vi "Add Package to Feed.vi"(4 "create new package destination folderpath if none exists (F)":bool, 6 "package destination folderpath":path, 7 "create new feed if none exists (F)":bool, 8 "error in":errorcluster, 9 "overwrite existing package (T)":bool=TRUE, 10 "package source filepath":path, 11 "feed folderpath in":path) -> (0 "error out":errorcluster, 2 "package destination filepath":path, 3 "feed folderpath out":path)   [LabVIEW 2014, in "NIPM_API.lvlib"]
doc: "Adds a package to a feed\n\nINPUT(s)\n<B>Feed folderpath</B>: Specifies the folder containing the feed\n\n<B>Package source filepath</B>: Specifies the source filepath of the package to be added to the feed\n\n<B>Create new feed if none exists</B>: If this input is set to TRUE, this VI will create a new feed if there are no existing feed files in the specified feed folderpath.\n\n<B>Overwrite existing package</B>: If this input is set to TRUE, this VI will copy the source package to the package destination folderpath and overwrite an existing package in the package destination folder if necessary.\n\n<B>Package destination folderpath</B>: If this input is left empty, this VI will default to using the feed folderpath as the package destination folderpath.\n\n<B>Create new package destination folder if none exists</B>: If this input is set to TRUE, this VI will create the package destination folder if it does not already exist.\n\nOUTPUT(s)\n<B>Feed folderpath out</B>: Outputs the specified feed folderpath\n\n<B>Package destination filepath</B>: Outputs the destination filepath of the package that was added to the feed"
uses:
  NIPM_API.lvlib
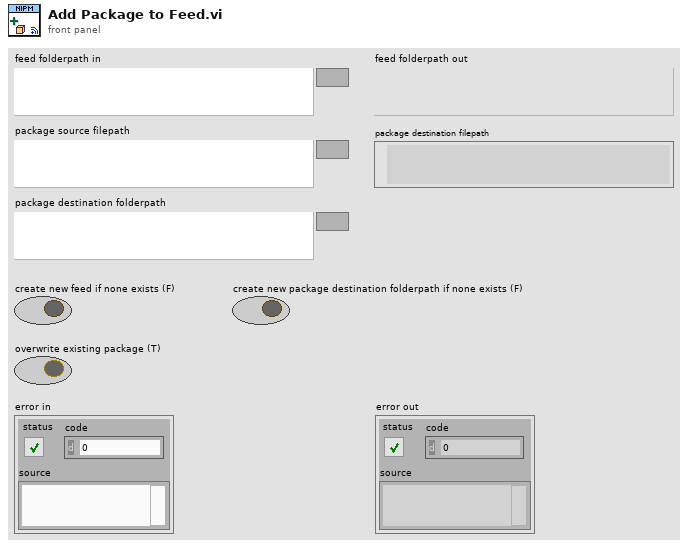
[diagram p1: front panel]
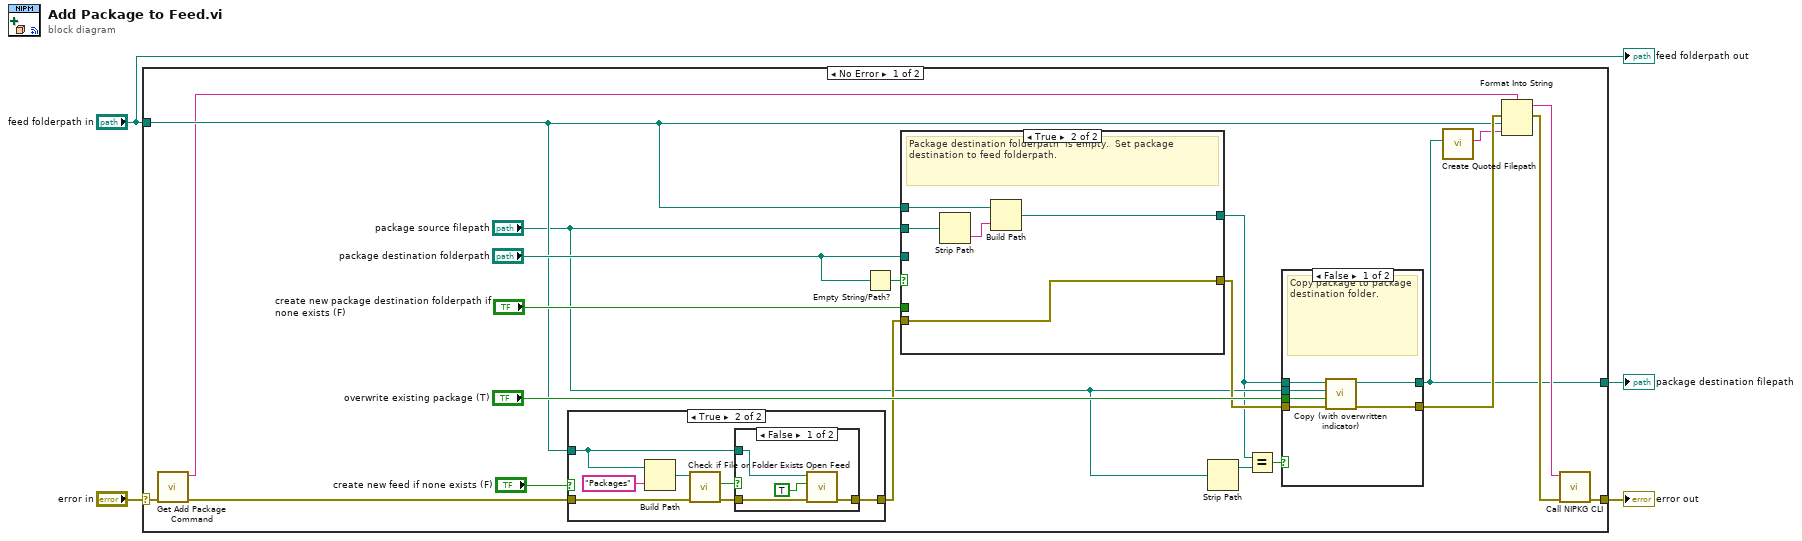
[diagram p0: block diagram]
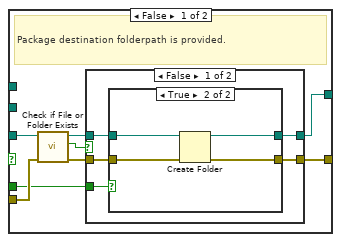
[diagram p3: hidden frame]
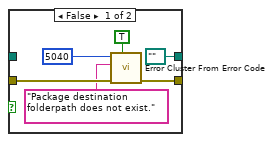
[diagram p4: hidden frame]
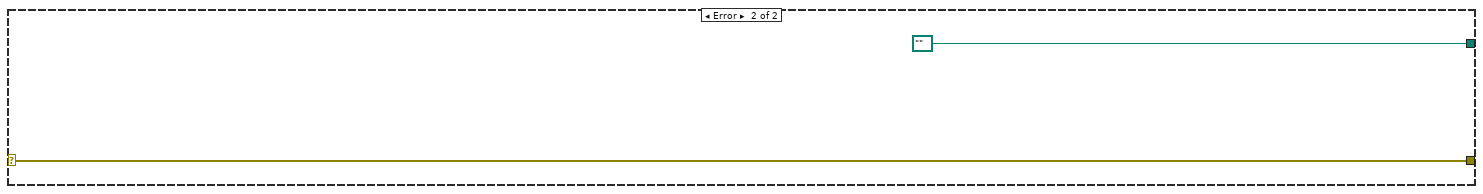
[diagram p8: hidden frame]
diagram:
  n1 = case shown="No Error" "error in" {
    selector: "error in" -> [w9 w78]
    tunnel: [w15 w78] -> w3
    tunnel: "feed folderpath in" -> [w14 _]
    tunnel: [w6 path "" ("new path")] -> w1
    frame No Error {
      n2 = call "Get Add Package Command.vi"("error in (no error)"=w9) -> ("error out"=w7:errorcluster, "Add Package to Feed Command"=w8:string)  [unwired: 9 in]
      n3 = case shown="True" "create new feed if none exists (F)" {
        tunnel: w7 -> [w64 w69]
        tunnel: [w64 w66] -> w19
        tunnel: w14 -> [_ w65]
        frame False {
        }
        frame True {
          n4 = Build Path(base path=w65, name or relative path="Packages") -> (appended path=w70:path)
          n5 = call <vilib>:"Check if File or Folder Exists.vi"("error in (no error)"=w69, "path"=w70) -> ("error out"=w67:errorcluster, "file or folder exists?"=w68:bool)  [unwired: 7 in, 1 out]
          n6 = case shown="False" w68 {
            tunnel: w67 -> [w75 w76]
            tunnel: [w74 w76] -> w66
            tunnel: w65 -> [w73 _]
            frame False {
              n7 = call "Open Feed.vi"("error in"=w75, "create feed if necessary (F)"=TRUE, "feed folderpath"=w73) -> ("error out"=w74:errorcluster)  [unwired: 6 in, 2 out]
            }
            frame True {
            }
          }
        }
      }
      n8 = Empty String/Path?(string/path="package destination folderpath") -> (empty?=w22:bool)
      n9 = case shown="True" w22 {
        tunnel: "package source filepath" -> [_ w63]
        tunnel: [w37 w61] -> w11
        tunnel: w14 -> [_ w60]
        tunnel: "package destination folderpath" -> [w41 _]
        tunnel: "create new package destination folderpath if none exists (F)" -> [w36 _]
        tunnel: w19 -> [w40 w59]
        tunnel: [w34 w59] -> w18
        frame False {
          # "Package destination folderpath is provided."
          n10 = call <vilib>:"Check if File or Folder Exists.vi"("error in (no error)"=w40, "path"=w41) -> ("error out"=w35:errorcluster, "file or folder exists?"=w39:bool, "dup path"=w38:path)  [unwired: 7 in]
          n11 = case shown="False" w39 {
            tunnel: w38 -> [w45 w58]
            tunnel: [w44 w58] -> w37
            tunnel: w36 -> [w46 _]
            tunnel: w35 -> [w43 w57]
            tunnel: [w42 w57] -> w34
            frame False {
              n12 = case shown="True" w46 {
                tunnel: w45 -> [_ w54]
                tunnel: [path "" ("dup path") w53] -> w44
                tunnel: w43 -> [w51 w56]
                tunnel: [w48 w55] -> w42
                frame False {
                  n13 = call <vilib>:"Error Cluster From Error Code.vi"("show call chain? (False)"=TRUE, "error in (no error)"=w51, "error message (\"\")"="Package destination folderpath does not exist.", "error code (0)"=5040) -> ("error out"=w48:errorcluster)  [unwired: 5 in]
                }
                frame True {
                  n14 = Create Folder(path (use dialog)=w54, error in=w56) -> (created path=w53:path, error out=w55:errorcluster)  [unwired: 1 in, 1 out]
                }
              }
            }
            frame True {
            }
          }
        }
        frame True {
          # "Package destination folderpath  is empty.  Set package destination to feed folderpath."
          n15 = Strip Path(path=w63) -> (name=w62:string)  [unwired: 1 out]
          n16 = Build Path(base path=w60, name or relative path=w62) -> (appended path=w61:path)
        }
      }
      n17 = Strip Path(path="package source filepath") -> (stripped path=w10:path)  [unwired: 1 out]
      n18 = Equal?(x=w11, y=w10) -> (x = y?=w12:bool)
      n19 = case shown="False" w12 {
        tunnel: "overwrite existing package (T)" -> [w31 _]
        tunnel: [w30 w32] -> w24
        tunnel: w18 -> [w29 w32]
        tunnel: [w28 w33] -> w6
        tunnel: w11 -> [w27 _]
        tunnel: "package source filepath" -> [w26 w33]
        frame False {
          # "Copy package to package destination folder."
          n20 = call "Copy (with overwritten indicator).vi"("error in (no error)"=w29, "overwrite (F)"=w31, "source filepath"=w26, "target folderpath"=w27) -> ("error out"=w30:errorcluster, "new path"=w28:path)  [unwired: 5 in, 1 out]
        }
        frame True {
          # "Package is already in the package destination folder. No need to copy file."
        }
      }
      n21 = call "Create Quoted Filepath.vi"("Path"=w6) -> ("Quoted Path String"=w5:string)  [unwired: 10 in]
      n22 = Format Into String(format string=w8, error in=w24, w14, w5) -> (resulting string=w17:string, error out=w16:errorcluster)  [unwired: 1 in]
      n23 = call "Call NIPKG CLI.vi"("error in (no error)"=w16, "command"=w17) -> ("error out"=w15:errorcluster)  [unwired: 8 in, 1 out]
    }
    frame Error {
    }
  }
  "error out" <- w3
  "package destination filepath" <- w1
  "feed folderpath out" <- "feed folderpath in"
